vi "Check if Calibration valid for current parameters.vi"(11 "System Information Cluster":T1) -> (1 "Calibration Not Required?":bool, 2 "Current Calibration Key":string, 3 "Calibration Valid?":bool)   [LabVIEW 2012]
uses:
  Custom Controls and Typedefs/SciScan System Information Cluster.ctl
  <vilib>/Utility/config.llb/NI_LVConfig.lvlib
  GFG/GFG library.lvlib
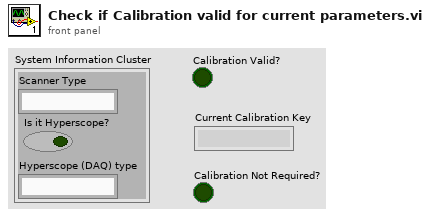
[diagram p1: front panel]
types:
  T1 = typedef "SciScan System Information Cluster.ctl" = cluster{"Scanner Type":string, "Is it Hyperscope?":bool, "Hyperscope (DAQ) type":string}
  T2 = typedef "NI_LVConfig.lvlib/Config Data RefNum.ctl" = refnum<k1>
  T3 = typedef "Calibration Key Param structure.ctl" = cluster{"GFG Variable Name":string, "Data Type":T4, "Value":variant}
  T4 = typedef "VariantType.lvlib/Type.ctl" = enum8{"Invalid Type", "Void", "I8", "I16", "I32", "I64", "U8", "U16", "U32", "U64", "Single Float", "Double Float", "Extended Float", "Single Complex", "Double Complex", "Extended Complex", "Enum U8", "Enum U16", "Enum U32", "Enum U64", "Single Float With Unit", "Double Float With Unit", "Extended Float With Unit", "Single Complex with Unit", "Double Complex with Unit", "Extended Complex with Unit", "Boolean", "String", "Path", "Picture", "Tag", "Array", "Cluster", "Variant", "LV Variant", "Waveform", "Timestamp", "Digital Waveform", "Digital Data", "ExpressData", "Refnum", "External Data", "VI", "Poly VI", "LabVIEW Class Instance", "Fixed Point"}
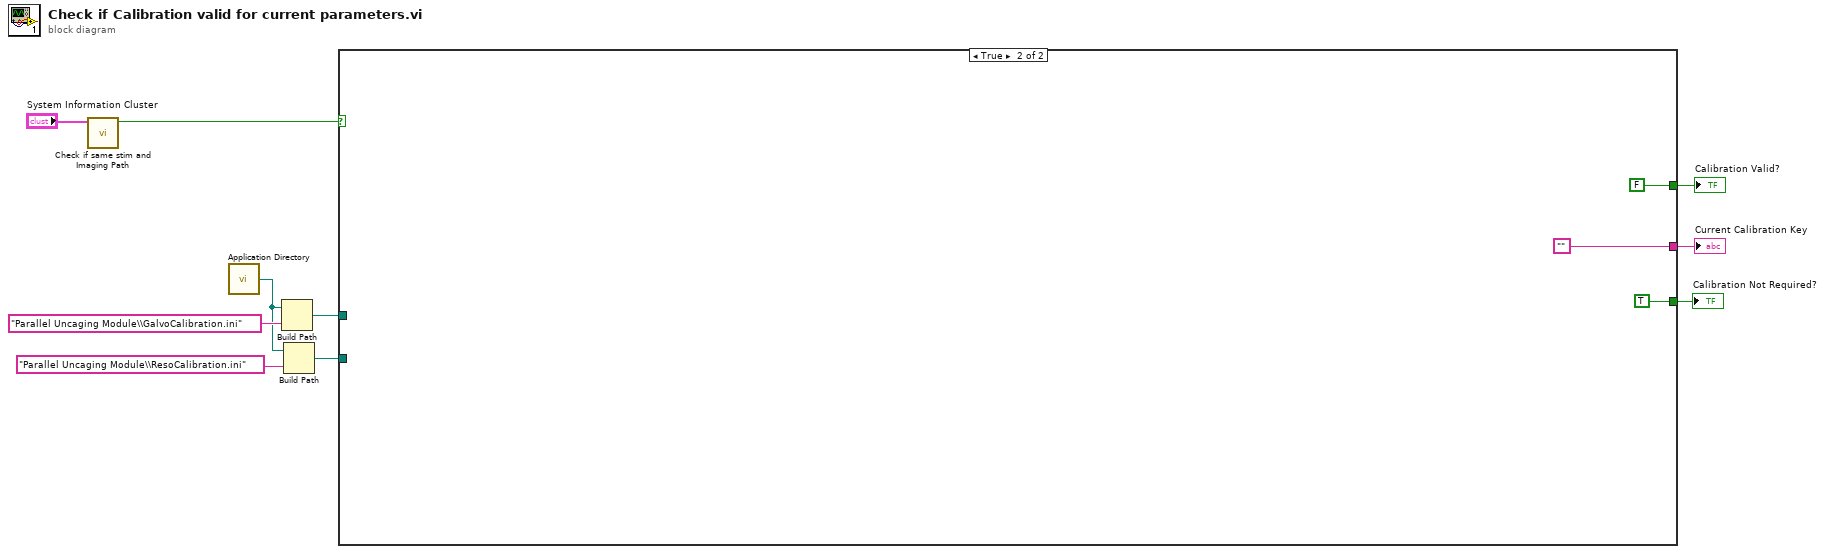
[diagram p0: block diagram]
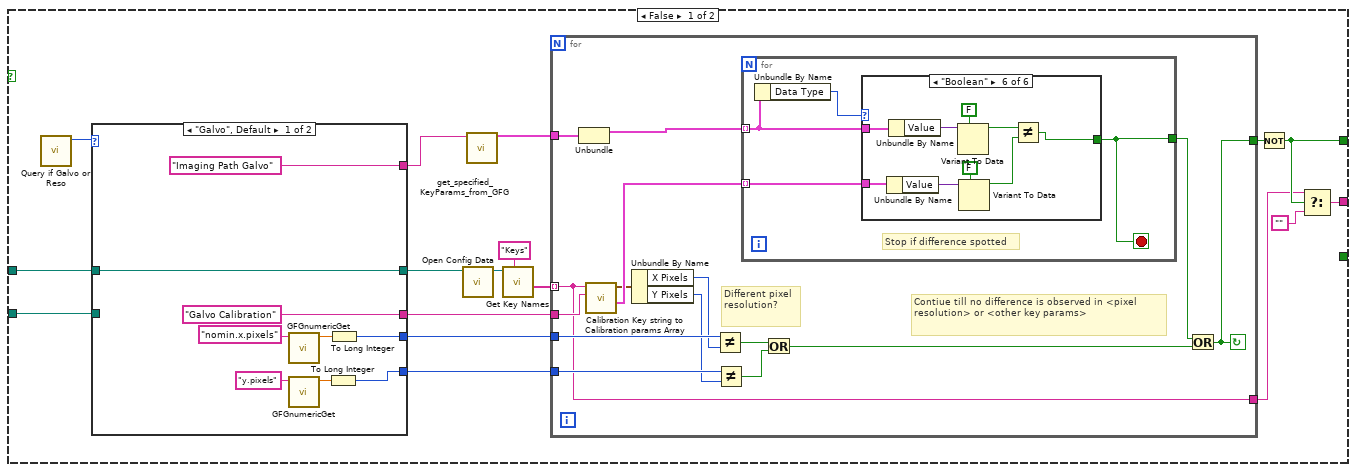
[diagram p2: hidden frame]
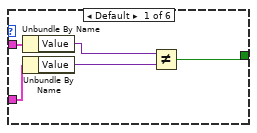
[diagram p3: hidden frame]
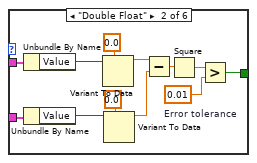
[diagram p4: hidden frame]
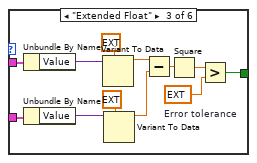
[diagram p5: hidden frame]
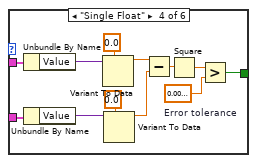
[diagram p6: hidden frame]
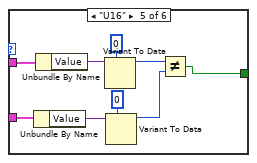
[diagram p7: hidden frame]
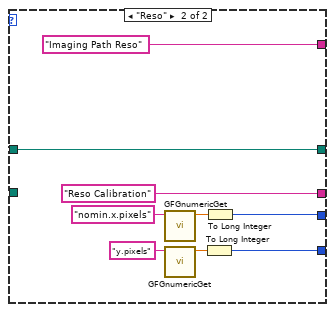
[diagram p8: hidden frame]
diagram:
  n1 = call "Check if same stim and Imaging Path.vi"("System Information Cluster"="System Information Cluster") -> ("Boolean"=w9:bool)  [unwired: 10 in]
  n2 = call <vilib>:"Application Directory.vi"() -> ("Application Directory"=w7:path)
  n3 = Build Path(base path=w7, name or relative path="Parallel Uncaging Module\\GalvoCalibration.ini") -> (appended path=w5:path)
  n4 = Build Path(base path=w7, name or relative path="Parallel Uncaging Module\\ResoCalibration.ini") -> (appended path=w4:path)
  n5 = case shown="True" w9 {
    tunnel: w5 -> [w26 _]
    tunnel: w4 -> [w25 _]
    tunnel: [w16 FALSE] -> w3
    tunnel: [w13 ""] -> w2
    tunnel: [_ TRUE] -> w1
    frame False {
      n6 = call "Query if Galvo or Reso.vi"() -> ("System Type"=w27:enum16{"Galvo", "Reso"})  [unwired: 10 in, 1 out]
      n7 = case shown="\"Galvo\", Default" w27 {
        tunnel: w26 -> [w113 _]
        tunnel: w25 -> [_ w122]
        tunnel: ["Imaging Path Galvo" ("Key Parameter Type") "Imaging Path Reso" ("Key Parameter Type")] -> w24
        tunnel: [w113 w122] -> w23
        tunnel: ["Galvo Calibration" ("section") "Reso Calibration" ("section")] -> w19
        tunnel: [w111 w116] -> w12
        tunnel: [w110 w115] -> w11
        frame "Galvo", Default {
          n8 = call "GFGnumericGet.vi"("Variable Name in"="nomin.x.pixels") -> ("Numeric"=w107:dbl)  [unwired: 8 in, 2 out]
          n9 = call "GFGnumericGet.vi"("Variable Name in"="y.pixels") -> ("Numeric"=w106:dbl)  [unwired: 8 in, 2 out]
          n10 = To Long Integer(number=w106) -> (32bit integer=w110:i32)
          n11 = To Long Integer(number=w107) -> (32bit integer=w111:i32)
        }
        frame "Reso" {
          n12 = call "GFGnumericGet.vi"("Variable Name in"="nomin.x.pixels") -> ("Numeric"=w119:dbl)  [unwired: 8 in, 2 out]
          n13 = call "GFGnumericGet.vi"("Variable Name in"="y.pixels") -> ("Numeric"=w120:dbl)  [unwired: 8 in, 2 out]
          n14 = To Long Integer(number=w120) -> (32bit integer=w115:i32)
          n15 = To Long Integer(number=w119) -> (32bit integer=w116:i32)
        }
      }
      n16 = call <vilib>:"Open Config Data.vi"("configuration file path"=w23) -> ("refnum"=w22:T2)  [unwired: 8 in, 2 out]
      n17 = call "get_specified_KeyParams_from_GFG.vi"("Key Parameter Type"=w24) -> ("Requested Key Parameters OUT"=w18:cluster{T3[], string})  [unwired: 10 in]
      n18 = call <vilib>:"Get Key Names.vi"("section"="Keys", "refnum"=w22) -> ("key names"=w20:string[])  [unwired: 6 in, 3 out]
      n19 = for {
        tunnel: w20 -> [w28] mode=indexing
        tunnel: w19 -> [w42]
        tunnel: w18 -> [w41]
        tunnel: [w29] -> w17
        tunnel: w12 -> [w37]
        tunnel: w11 -> [w35]
        tunnel: [w28] -> w15
        stop <- w29 continue-if-true
        # "Different pixel resolution?"
        # "Contiue till no difference is observed in <pixel resolution> or <other key params>"
        n20 = Unbundle(w41) -> (w40:T3[])  [unwired: 1 out]
        n21 = call "Calibration Key string to Calibration params Array.vi"("Calibration Type"=w42, "Key String IN"=w28) -> ("Imaging (Galvo/Reso) Key Array"=w39:T3[], "Image Pixels OUT"=w38:cluster{"X Pixels":i32, "Y Pixels":i32})  [unwired: 7 in, 1 out]
        n22 = Unbundle By Name(w38) -> ("X Pixels"=w36:i32, "Y Pixels"=w34:i32)
        n23 = Not Equal?(x=w37, y=w36) -> (x != y?=w33:bool)
        n24 = Not Equal?(x=w35, y=w34) -> (x != y?=w32:bool)
        n25 = for {
          tunnel: w40 -> [w44] mode=indexing
          tunnel: w39 -> [w46] mode=indexing
          tunnel: [w45] -> w31
          stop <- w45 stop-if-true
          # "Stop if difference spotted"
          n26 = Unbundle By Name(w44) -> ("Data Type"=w43:T4)
          n27 = case shown="\"Boolean\"" w43 {
            tunnel: w46 -> [w51 w62 w74 w86 w95 w104]
            tunnel: [w48 w52 w64 w76 w88 w99] -> w45
            tunnel: w44 -> [w47 w63 w75 w87 w96 w105]
            frame Default {
              n28 = Unbundle By Name(w47) -> ("Value"=w50:variant)
              n29 = Unbundle By Name(w51) -> ("Value"=w49:variant)
              n30 = Not Equal?(x=w50, y=w49) -> (x != y?=w48:bool)
            }
            frame "Double Float" {
              w54 = 0.01  # Error tolerance
              n31 = Unbundle By Name(w63) -> ("Value"=w61:variant)
              n32 = Unbundle By Name(w62) -> ("Value"=w58:variant)
              n33 = Variant To Data(type=0.0, Variant=w61) -> (data=w57:dbl)  [unwired: 1 in, 1 out]
              n34 = Variant To Data(type=0.0, Variant=w58) -> (data=w56:dbl)  [unwired: 1 in, 1 out]
              n35 = Subtract(x=w57, y=w56) -> (x-y=w55:dbl)
              n36 = Square(x=w55) -> (x^2=w53:dbl)
              n37 = Greater?(x=w53, y=w54) -> (0:w52:bool)
            }
            frame "Extended Float" {
              w66 = ext 0.01  # Error tolerance
              n38 = Unbundle By Name(w75) -> ("Value"=w73:variant)
              n39 = Unbundle By Name(w74) -> ("Value"=w70:variant)
              n40 = Variant To Data(type=ext 0.0, Variant=w73) -> (data=w69:ext)  [unwired: 1 in, 1 out]
              n41 = Variant To Data(type=ext 0.0, Variant=w70) -> (data=w68:ext)  [unwired: 1 in, 1 out]
              n42 = Subtract(x=w69, y=w68) -> (x-y=w67:ext)
              n43 = Square(x=w67) -> (x^2=w65:ext)
              n44 = Greater?(x=w65, y=w66) -> (0:w64:bool)
            }
            frame "Single Float" {
              w78 = sgl 0.01  # Error tolerance
              n45 = Unbundle By Name(w87) -> ("Value"=w85:variant)
              n46 = Unbundle By Name(w86) -> ("Value"=w82:variant)
              n47 = Variant To Data(type=sgl 0.0, Variant=w85) -> (data=w81:sgl)  [unwired: 1 in, 1 out]
              n48 = Variant To Data(type=sgl 0.0, Variant=w82) -> (data=w80:sgl)  [unwired: 1 in, 1 out]
              n49 = Subtract(x=w81, y=w80) -> (x-y=w79:sgl)
              n50 = Square(x=w79) -> (x^2=w77:sgl)
              n51 = Greater?(x=w77, y=w78) -> (0:w76:bool)
            }
            frame "U16" {
              n52 = Unbundle By Name(w95) -> ("Value"=w91:variant)
              n53 = Unbundle By Name(w96) -> ("Value"=w93:variant)
              n54 = Variant To Data(type=u16 0, Variant=w93) -> (data=w90:u16)  [unwired: 1 in, 1 out]
              n55 = Variant To Data(type=u16 0, Variant=w91) -> (data=w89:u16)  [unwired: 1 in, 1 out]
              n56 = Not Equal?(x=w90, y=w89) -> (x != y?=w88:bool)
            }
            frame "Boolean" {
              n57 = Unbundle By Name(w104) -> ("Value"=w102:variant)
              n58 = Unbundle By Name(w105) -> ("Value"=w103:variant)
              n59 = Variant To Data(type=FALSE, Variant=w103) -> (data=w101:bool)  [unwired: 1 in, 1 out]
              n60 = Variant To Data(type=FALSE, Variant=w102) -> (data=w100:bool)  [unwired: 1 in, 1 out]
              n61 = Not Equal?(x=w101, y=w100) -> (x != y?=w99:bool)
            }
          }
        }
        n62 = Or(x=w33, y=w32) -> (x .or. y?=w30:bool)
        n63 = Or(x=w31, y=w30) -> (x .or. y?=w29:bool)
      }
      n64 = Not(x=w17) -> (.not. x?=w16:bool)
      n65 = Select(t=w15, s=w16, f="") -> (s? t:f=w13:string)
    }
    frame True {
    }
  }
  "Calibration Valid?" <- w3
  "Current Calibration Key" <- w2
  "Calibration Not Required?" <- w1
